vi "Profiler tester.vi"() -> ()   [LabVIEW 2014]
uses:
  Max profiles.ctl
  TimeSegments.ctl
  TimeSegment.ctl
panel:
  in  "Which solver":bool
  out "Determinted":dbl
  in  "initalVelocity":dbl format="%#_13g"
  in  "initalAccel":dbl format="%#_13g"
  out "output variable":dbl
  out "Acceleration Graph 3":cluster{"X":dbl, "Y":dbl}[](graph)
  out "Velocity Graph 2":cluster{"X":dbl, "Y":dbl}[](graph)
  out "TimeSegments":T1
  out "Position Graph":cluster{"X":dbl, "Y":dbl}[](graph)
  in  "Seconds to graph":dbl=10.0 format="%#_13g"
  in  "Max profiles":T3={"Max jerk"=100.0, "Max acceleration"=10.0, "Max Velocity"=10.0}
  in  "Distance to go":dbl=10.0 format="%#_13g"
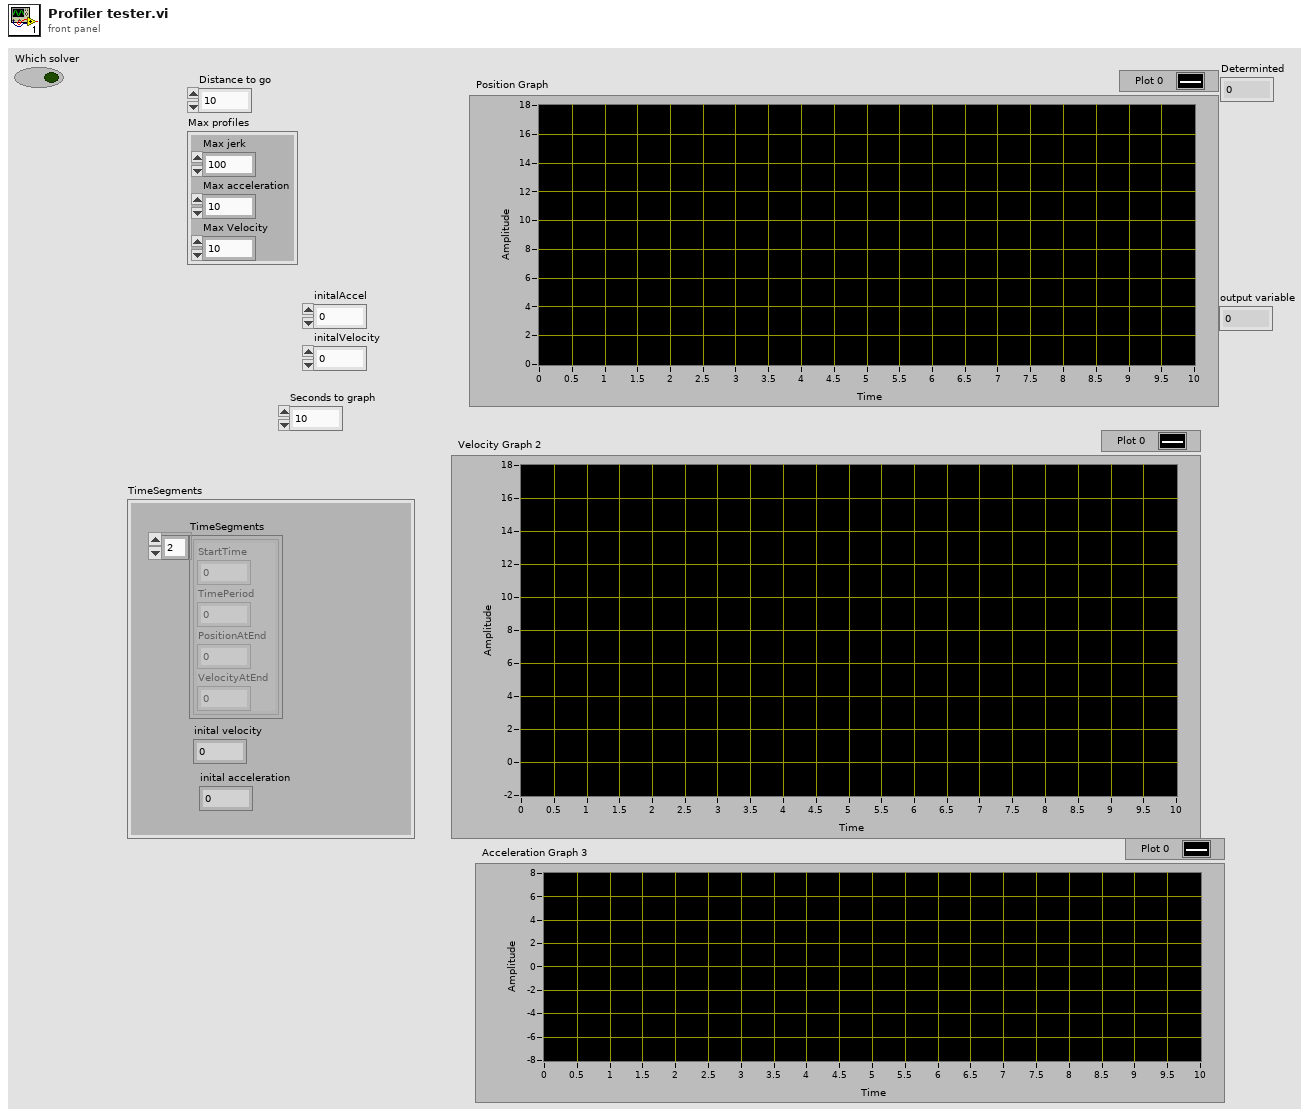
[diagram p1: front panel]
types:
  T1 = typedef "TimeSegments.ctl" = cluster{"TimeSegments":T2[], "inital velocity":dbl, "inital acceleration":dbl}
  T2 = typedef "TimeSegment.ctl" = cluster{"StartTime":dbl, "TimePeriod":dbl, "PositionAtEnd":dbl, "VelocityAtEnd":dbl}
  T3 = typedef "Max profiles.ctl" = cluster{"Max jerk":dbl, "Max acceleration":dbl, "Max Velocity":dbl}
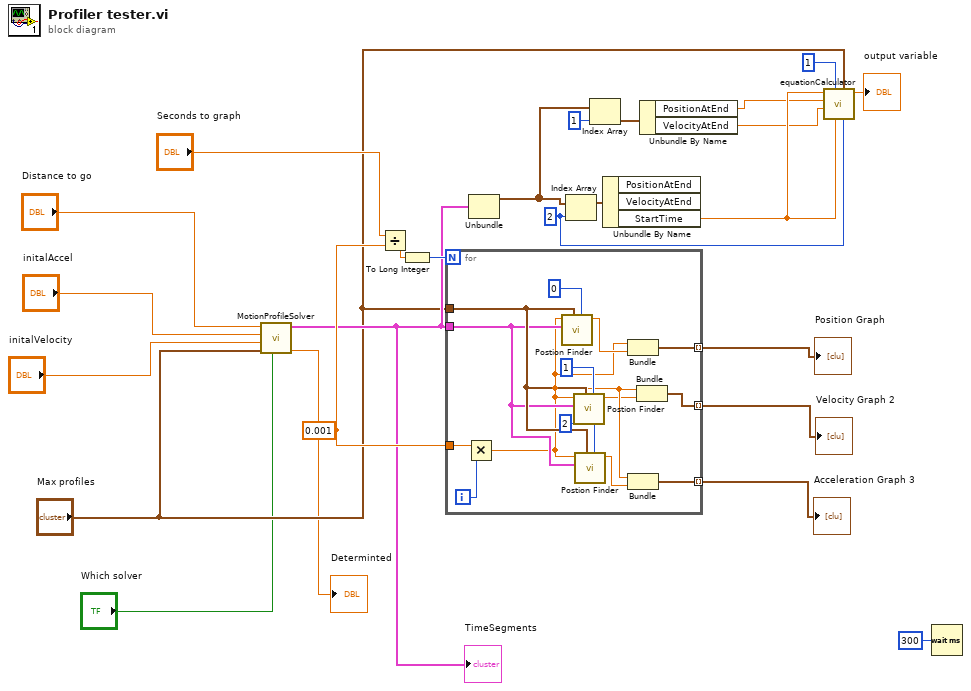
[diagram p0: block diagram]
diagram:
  w12 = 2 ("index")
  w21 = 0.001
  n1 = call "MotionProfileSolver.vi"("Which solver"="Which solver", "Max profiles"="Max profiles", "initalVelocity"="initalVelocity", "initalAccel"="initalAccel", "Distance to go"="Distance to go") -> ("Determinted"=→"Determinted":dbl, "TimeSegments"=w16:T1)  [unwired: 5 in]
  "TimeSegments" <- w16
  n2 = Divide(x="Seconds to graph", y=w21) -> (x/y=w22:dbl)
  n3 = To Long Integer(number=w22) -> (32bit integer=w23:i32)
  n4 = for {
    N: w23 -> [_]
    tunnel: w16 -> [w32]
    tunnel: [w38] -> w20 mode=indexing
    tunnel: "Max profiles" -> [w33]
    tunnel: w21 -> [w37]
    tunnel: [w28] -> w19 mode=indexing
    tunnel: [w27] -> w18 mode=indexing
    i -> [w39]
    n5 = Multiply(x=w37, y=w39) -> (x*y=w30:dbl)
    n6 = call "Postion Finder.vi"("derivitave"=i8 0, "Max profiles"=w33, "TimeSegments"=w32, "time"=w30) -> ("Motion Profiler Setpoint"=w36:dbl)  [unwired: 7 in]
    n7 = call "Postion Finder.vi"("derivitave"=i8 1, "Max profiles"=w33, "TimeSegments"=w32, "time"=w30) -> ("Motion Profiler Setpoint"=w29:dbl)  [unwired: 7 in]
    n8 = call "Postion Finder.vi"("derivitave"=i8 2, "Max profiles"=w33, "TimeSegments"=w32, "time"=w30) -> ("Motion Profiler Setpoint"=w26:dbl)  [unwired: 7 in]
    n9 = Bundle(w30, "Motion Profiler Setpoint"=w36) -> (w38:cluster{dbl, "Motion Profiler Setpoint":dbl})  [unwired: 1 in]
    n10 = Bundle(w30, "Motion Profiler Setpoint"=w26) -> (w27:cluster{dbl, "Motion Profiler Setpoint":dbl})  [unwired: 1 in]
    n11 = Bundle(w30, "Motion Profiler Setpoint"=w29) -> (w28:cluster{dbl, "Motion Profiler Setpoint":dbl})  [unwired: 1 in]
  }
  "Position Graph" <- w20
  "Velocity Graph 2" <- w19
  "Acceleration Graph 3" <- w18
  n12 = Unbundle(w16) -> ("TimeSegments"=w10:T2[])  [unwired: 2 out]
  n13 = Index Array(array=w10, index=w12) -> (element=w17:T2)
  n14 = Index Array(array=w10, index=1) -> (element=w8:T2)
  n15 = Unbundle By Name(w17) -> ("StartTime"=w13:dbl)  [unwired: 2 out]
  n16 = Unbundle By Name(w8) -> ("PositionAtEnd"=w7:dbl, "VelocityAtEnd"=w6:dbl)
  n17 = call "equationCalculator.vi"("Time Segment"=w12, "Max profiles"="Max profiles", "startOfTimePeriod"=w13, "derivitave"=i8 1, "vInital"=w6, "xInital"=w7, "currentTime"=w13) -> ("output variable"=→"output variable":dbl)  [unwired: 4 in]
  n18 = Wait (ms)(milliseconds to wait=u32 300) -> ()  [unwired: 1 out]
